vi "MSTSoftwareBin_Final.vi"() -> ()   [LabVIEW 2012]
uses:
  <vilib>/addons/database/Auxilliary.llb/DB Tools Cursor Type.ctl
  <vilib>/Utility/NIReport.llb/NI_report.lvclass
  <vilib>/addons/database/Connection.llb/DB Tools Open Connec (Path).vi
  <vilib>/addons/database/Connection.llb/Conn Execute.vi
  <vilib>/addons/database/Recordset.llb/Rec Fetch Recordset Data (R).vi
  <vilib>/addons/database/Recordset.llb/Rec Destroy - Connection.vi
  <vilib>/Utility/NIReport.llb/Append Text Table to Report (wrap).vi
  <vilib>/addons/database/_DB Variant To Data/Database Variant To Data.xnode
  <vilib>/addons/database/NI_Database_API.lvlib
  <vilib>/Utility/NIReport.llb/Excel/NI_Excel.lvclass
panel:
  out "error out":errorcluster
  out "recordset data":variant[][](array[variant])
  out "data":string
  out "appended array":string[](array[string])
  in  "Report Template":path=path "O:/Monitor/Report/MSTsoftBin.xls"
  out "Row Headers":string[](array[string])
  out "error out 2":errorcluster
  out "concatenated string":string
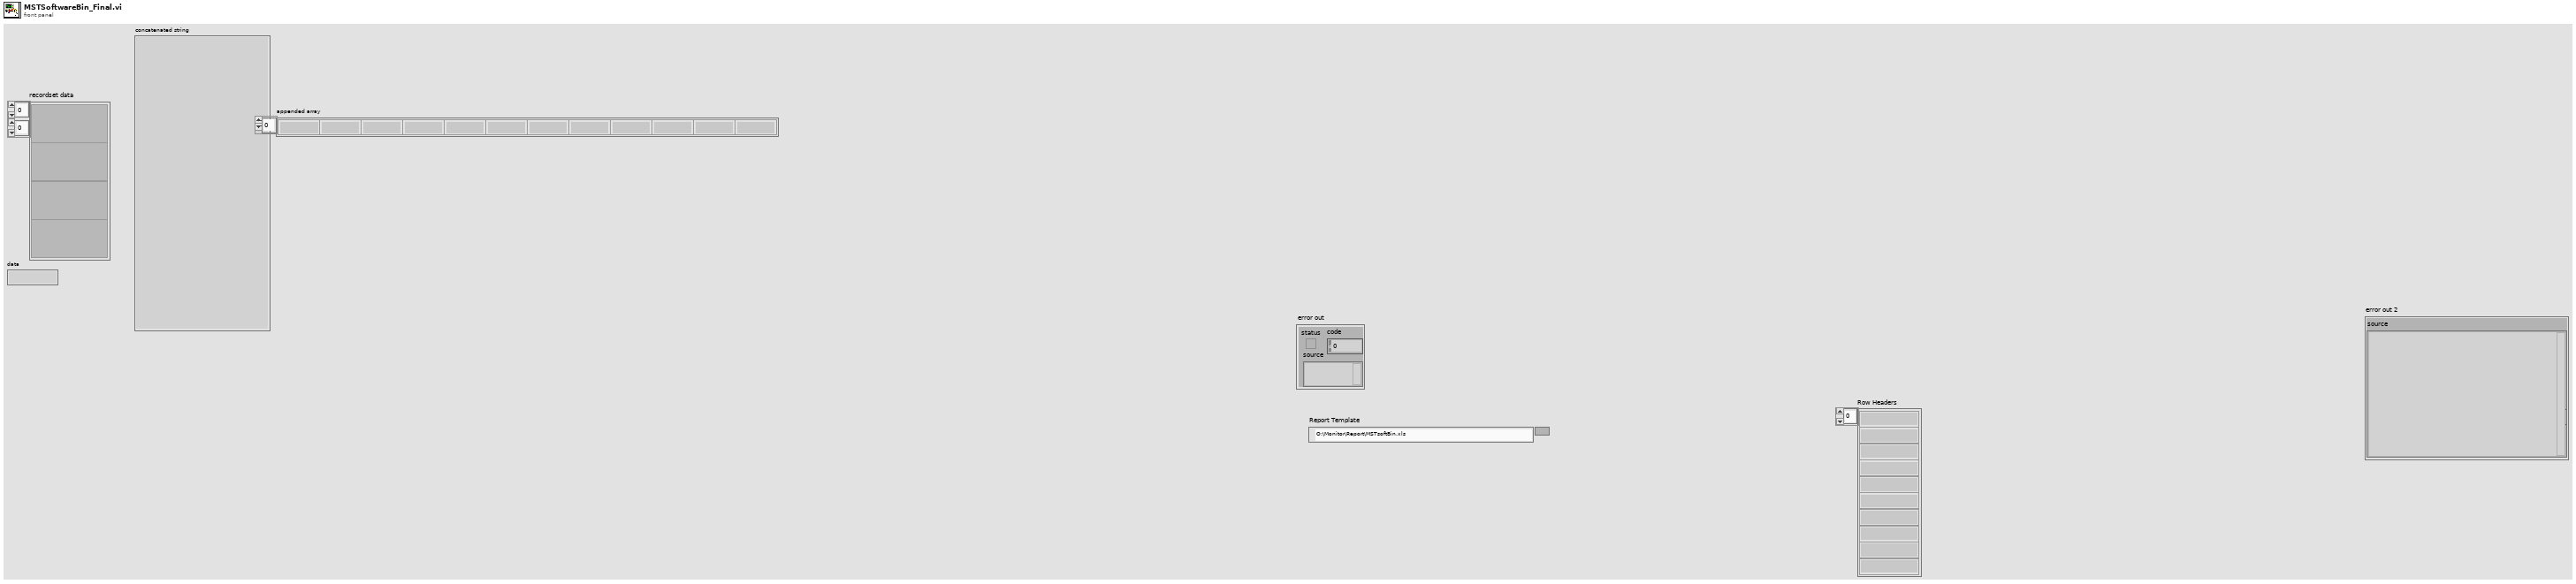
[diagram p1: front panel]
types:
  T1 = typedef "NI_Database_API.lvlib/DB Tools Cursor Type.ctl" = enum16{"forward-only", "keyset", "dynamic", "static"}
  T2 = enum16{"Standard Report", "HTML", "Word", "Excel"}
  T3 = typedef "NI_Database_API.lvlib/Conn ObjectReference.ctl" = refnum<k1>
  T4 = typedef "NI_Database_API.lvlib/Rec ObjectReference.ctl" = refnum<k1>
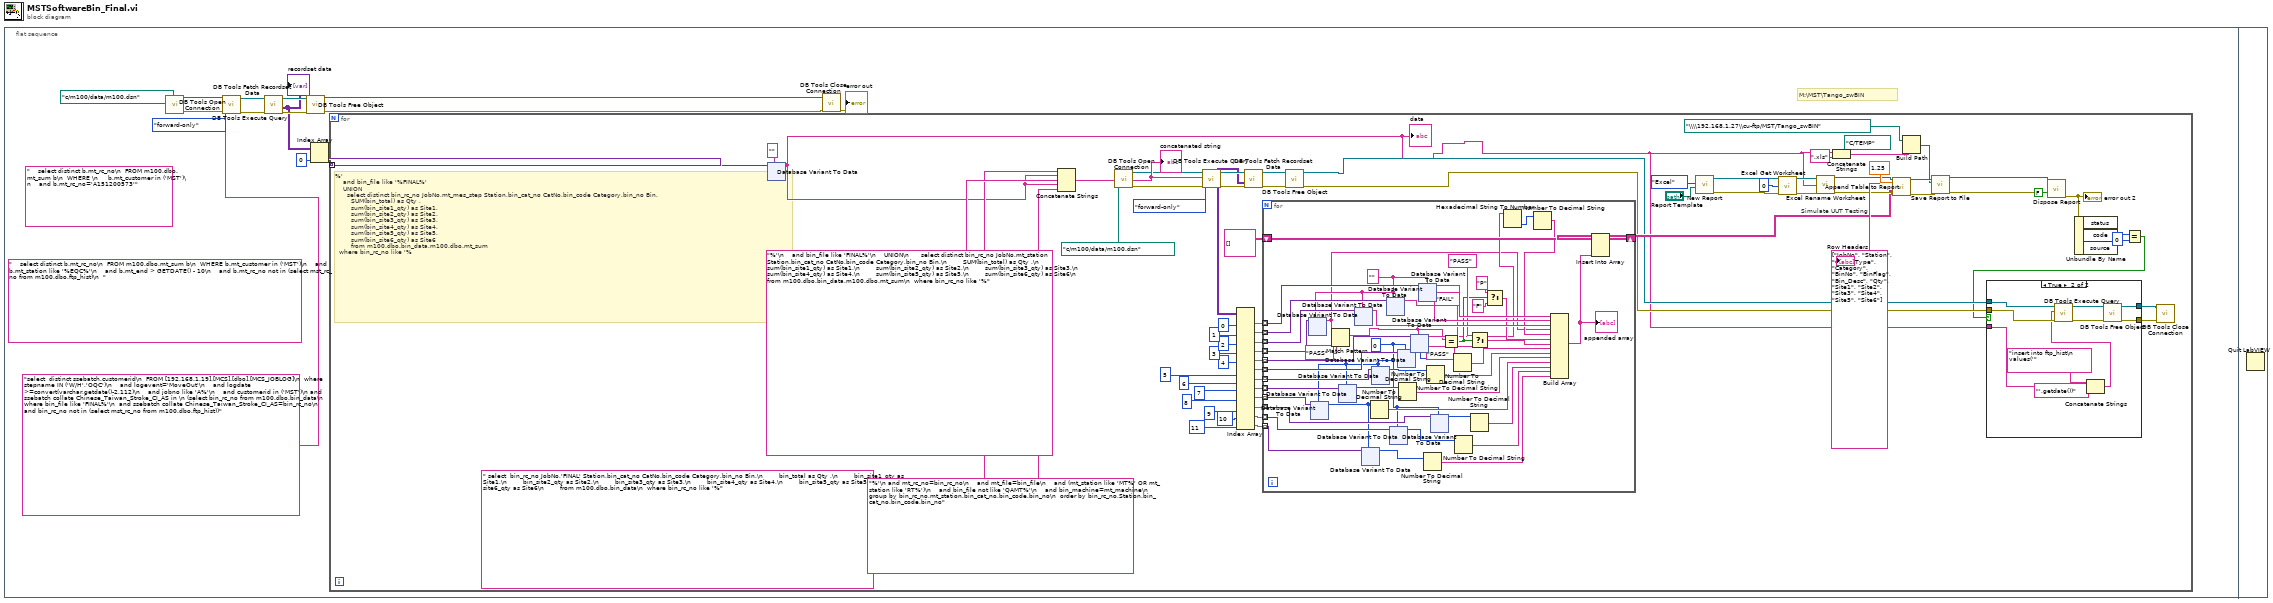
[diagram p0: block diagram]
diagram:
  n1 = flat-sequence {
    frame #0 {
      (unwired) "    select distinct b.mt_rc_no\n  FROM m100.dbo.mt_sum b\n  WHERE b.mt_customer in ('MST')\n    and b.mt_station like '%EQC%'\n    and b.mt_end > GETDATE() - 10\n    and b.mt_rc_no not in (select mst_rc_no from m100.dbo.ftp_hist)\n  " ("SQL query")
      (unwired) "    select distinct b.mt_rc_no\n  FROM m100.dbo.mt_sum b\n  WHERE \n     b.mt_customer in ('MST')\n    and b.mt_rc_no='A151200573'" ("SQL query")
      # "M:\\MST\\Tango_swBIN"
      n2 = call-poly <vilib>:"DB Tools Open Connection.vi"("connection information"=path "c:/m100/data/m100.dsn") -> ("error out"=w12:errorcluster, "connection reference"=w15:T3)  [unwired: 7 in]
      n3 = call-poly <vilib>:"DB Tools Execute Query.vi"("error in (no error)"=w12, "cursor type"=DB_Tools_Cursor_Type."forward-only", "SQL query"="select  distinct ssebatch,customerid\n  FROM [192.168.1.19].[MCS].[dbo].[MCS_JOBLOG]\n  where  stepname IN ('W/H','OQC')\n    and logevent='MoveOut'\n    and logdate >=convert(varchar,getdate()-2,112)\n    and jobno like 'A%'\n    and customerid in ('MST')\n and ssebatch collate Chinese_Taiwan_Stroke_CI_AS in \n (select bin_rc_no from m100.dbo.bin_data\n  where bin_file like 'FINAL%'\n  and ssebatch collate Chinese_Taiwan_Stroke_CI_AS=bin_rc_no\n  and bin_rc_no not in (select mst_rc_no from m100.dbo.ftp_hist))", "connection reference"=w15) -> ("error out"=w11:errorcluster, "recordset reference"=w14:T4)  [unwired: 4 in]
      n4 = call-poly <vilib>:"DB Tools Fetch Recordset Data.vi"("error in (no error)"=w11, "recordset reference"=w14) -> ("error out"=w10:errorcluster, "recordset data"=w7:variant[][], "recordset reference out"=w13:T4)  [unwired: 3 in]
      "recordset data" <- w7
      n5 = call-poly <vilib>:"DB Tools Free Object.vi"("error in (no error)"=w10, "recordset reference"=w13) -> ("error out"=w3:errorcluster, "connection reference"=w4:T3)  [unwired: 8 in]
      n6 = Index Array(array=w7, index (col)=0 ("disabled index (col)")) -> (element=w5:variant[])  [unwired: 1 in]
      n7 = for {
        tunnel: w5 -> [w85] mode=indexing
        (unwired) path "C:/TEMP" ("base path")
        # "%'\n    and bin_file like '%FINAL%'\n    UNION\n      select distinct bin_rc_no JobNo,mt_mes_step Station,bin_cat_no CatNo,bin_code Category,bin_no Bin,\n        SUM(bin_total) as Qty ,\n        sum(bin_site1_qty) as Site1,\n        sum(bin_site2_qty) as Site2,\n        sum(bin_site3_qty) as Site3,\n        sum(bin_site4_qty) as Site4,\n        sum(bin_site5_qty) as Site5,\n        sum(bin_site6_qty) as Site6\n        from m100.dbo.bin_data,m100.dbo.mt_sum\n  where bin_rc_no like '%"
        # "Simulate UUT Testing"
        n8 = xnode "Database Variant To Data"("database variant"=w85, "type"="") -> ("data"=w17:string)  [unwired: 1 in, 1 out]
        "data" <- w17
        n9 = Concatenate Strings(" select  bin_rc_no JobNo,'FINAL' Station,bin_cat_no CatNo,bin_code Category,bin_no Bin,\n        bin_total as Qty ,\n        bin_site1_qty as Site1,\n        bin_site2_qty as Site2,\n        bin_site3_qty as Site3,\n        bin_site4_qty as Site4,\n        bin_site5_qty as Site5,\n        bin_site6_qty as Site6\n        from m100.dbo.bin_data\n  where bin_rc_no like '%" ("string"), w17, "%'\n    and bin_file like 'FINAL%'\n    UNION\n      select distinct bin_rc_no JobNo,mt_station Station,bin_cat_no CatNo,bin_code Category,bin_no Bin,\n        SUM(bin_total) as Qty ,\n        sum(bin_site1_qty) as Site1,\n        sum(bin_site2_qty) as Site2,\n        sum(bin_site3_qty) as Site3,\n        sum(bin_site4_qty) as Site4,\n        sum(bin_site5_qty) as Site5,\n        sum(bin_site6_qty) as Site6\n        from m100.dbo.bin_data,m100.dbo.mt_sum\n  where bin_rc_no like '%" ("string"), w17, "%'\n and mt_rc_no=bin_rc_no\n    and mt_file=bin_file\n    and (mt_station like 'MT%' OR mt_station like 'RT%')\n    and bin_file not like 'QAMT%'\n    and bin_machine=mt_machine\n  group by bin_rc_no,mt_station,bin_cat_no,bin_code,bin_no\n  order by bin_rc_no,Station,bin_cat_no,bin_code,bin_no" ("string")) -> (w76:string)
        "concatenated string" <- w76
        n10 = call-poly <vilib>:"DB Tools Open Connection.vi"("connection information"=path "c:/m100/data/m100.dsn") -> ("error out"=w22:errorcluster, "connection reference"=w23:T3)  [unwired: 7 in]
        n11 = call-poly <vilib>:"DB Tools Execute Query.vi"("error in (no error)"=w22, "cursor type"=DB_Tools_Cursor_Type."forward-only", "SQL query"=w76, "connection reference"=w23) -> ("error out"=w81:errorcluster, "recordset reference"=w83:T4)  [unwired: 4 in]
        n12 = call-poly <vilib>:"DB Tools Fetch Recordset Data.vi"("error in (no error)"=w81, "recordset reference"=w83) -> ("error out"=w80:errorcluster, "recordset data"=w75:variant[][], "recordset reference out"=w82:T4)  [unwired: 3 in]
        n13 = Index Array(array=w75, index (col) #1=0 ("disabled index (col)"), index (col) #2=1 ("index (col)"), index (col) #3=2 ("index (col)"), index (col) #4=3 ("index (col)"), index (col) #5=4 ("index (col)"), index (col) #6=5 ("index (col)"), index (col) #7=6 ("index (col)"), index (col) #8=7 ("index (col)"), index (col) #9=8 ("index (col)"), index (col) #10=9 ("index (col)"), index (col) #11=10 ("index (col)"), index (col) #12=11 ("index (col)")) -> (element #1=w64:variant[], element #2=w63:variant[], element #3=w62:variant[], element #4=w61:variant[], element #5=w60:variant[], element #6=w59:variant[], element #7=w58:variant[], element #8=w57:variant[], element #9=w56:variant[], element #10=w55:variant[], element #11=w52:variant[], element #12=w51:variant[])  [unwired: 12 in]
        n14 = for {
          tunnel: w64 -> [w145] mode=indexing
          tunnel: w63 -> [w144] mode=indexing
          tunnel: w62 -> [w143] mode=indexing
          tunnel: w61 -> [w142] mode=indexing
          tunnel: w60 -> [w141] mode=indexing
          tunnel: w59 -> [w140] mode=indexing
          tunnel: w58 -> [w139] mode=indexing
          tunnel: w57 -> [w138] mode=indexing
          tunnel: w56 -> [w137] mode=indexing
          tunnel: w55 -> [w136] mode=indexing
          tunnel: w52 -> [w127] mode=indexing
          tunnel: w51 -> [w126] mode=indexing
          shift-right: [w121] -> w38
          shift-left: string[][] [] ("array") -> [w120]
          w112 = 0
          w135 = ""
          n15 = xnode "Database Variant To Data"("database variant"=w142, "type"=w135) -> ("data"=w100:string)  [unwired: 1 in, 1 out]
          n16 = xnode "Database Variant To Data"("database variant"=w137, "type"=w112) -> ("data"=w124:i32)  [unwired: 1 in, 1 out]
          n17 = Match Pattern(string=w100, regular expression="PASS") -> (match substring=w98:string)  [unwired: 1 in, 3 out]
          n18 = xnode "Database Variant To Data"("database variant"=w138, "type"=w112) -> ("data"=w129:i32)  [unwired: 1 in, 1 out]
          n19 = xnode "Database Variant To Data"("database variant"=w143, "type"=w135) -> ("data"=w132:string)  [unwired: 1 in, 1 out]
          n20 = xnode "Database Variant To Data"("database variant"=w126, "type"=w124) -> ("data"=w125:i32)  [unwired: 1 in, 1 out]
          n21 = Number To Decimal String(number=w124) -> (decimal integer string=w116:string)  [unwired: 1 in]
          n22 = xnode "Database Variant To Data"("database variant"=w139, "type"=w112) -> ("data"=w130:i32)  [unwired: 1 in, 1 out]
          n23 = xnode "Database Variant To Data"("database variant"=w144, "type"=w135) -> ("data"=w133:string)  [unwired: 1 in, 1 out]
          n24 = xnode "Database Variant To Data"("database variant"=w127, "type"=w112) -> ("data"=w123:i32)  [unwired: 1 in, 1 out]
          n25 = xnode "Database Variant To Data"("database variant"=w140, "type"=w112) -> ("data"=w131:i32)  [unwired: 1 in, 1 out]
          n26 = Number To Decimal String(number=w129) -> (decimal integer string=w115:string)  [unwired: 1 in]
          n27 = xnode "Database Variant To Data"("database variant"=w141, "type"=w98) -> ("data"=w102:string)  [unwired: 1 in, 1 out]
          n28 = xnode "Database Variant To Data"("database variant"=w145, "type"=w135) -> ("data"=w134:string)  [unwired: 1 in, 1 out]
          n29 = Number To Decimal String(number=w125) -> (decimal integer string=w119:string)  [unwired: 1 in]
          n30 = Number To Decimal String(number=w130) -> (decimal integer string=w114:string)  [unwired: 1 in]
          n31 = xnode "Database Variant To Data"("database variant"=w136, "type"=w112) -> ("data"=w128:i32)  [unwired: 1 in, 1 out]
          n32 = Equal?(x=w98, y="PASS") -> (x = y?=w108:bool)
          n33 = Number To Decimal String(number=w131) -> (decimal integer string=w113:string)  [unwired: 1 in]
          n34 = Number To Decimal String(number=w123) -> (decimal integer string=w118:string)  [unwired: 1 in]
          n35 = Number To Decimal String(number=w128) -> (decimal integer string=w117:string)  [unwired: 1 in]
          n36 = Select(t="PASS", s=w108, f="FAIL") -> (s? t:f=w109:string)
          n37 = Select(t="P", s=w108, f="F") -> (s? t:f=w105:string)
          n38 = Hexadecimal String To Number(string=w102) -> (number=w103:u32)  [unwired: 2 in, 1 out]
          n39 = Number To Decimal String(number=w103) -> (decimal integer string=w101:string)  [unwired: 1 in]
          n40 = Build Array(w134, w133, w132, w100, w101, w105, w109, w113, w114, w115, w116, w117, w118, w119) -> (w122:string[])
          "appended array" <- w122
          n41 = Insert Into Array(array=w120, new element=w122) -> (w121:string[][])  [unwired: 2 in]
        }
        n42 = call-poly <vilib>:"DB Tools Free Object.vi"("error in (no error)"=w80, "recordset reference"=w82) -> ("error out"=w27:errorcluster, "connection reference"=w28:T3)  [unwired: 8 in]
        n43 = call <vilib>:"New Report.vi"("report type"=T2."Excel" ("Report Type"), "template (empty)"="Report Template") -> ("report out"=w45:refnum<class "NI_report.lvclass">, "error out"=w44:errorcluster)  [unwired: 12 in]
        n44 = call <vilib>:"Excel Get Worksheet.vi"("report in"=w45, "worksheet index (0)"=0, "error in (no error)"=w44) -> ("report out"=w42:refnum<class "NI_report.lvclass">, "error out"=w40:errorcluster)  [unwired: 11 in]
        n45 = call <vilib>:"Excel Rename Worksheet.vi"("report in"=w42, "worksheet name (\"\")"=w17, "error in (no error)"=w40) -> ("report out"=w41:refnum<class "NI_report.lvclass">, "error out"=w39:errorcluster)  [unwired: 11 in]
        n46 = Concatenate Strings(w17, ".xls" ("string")) -> (w31:string)
        n47 = call-poly <vilib>:"Append Table to Report.vi"("report in"=w41, "column width (1)"=1.25, "column headers"=string[] ["JobNo", "Station", "CatNo Type", "Category", "BinNo", "BinFlag", "Bin_Desc", "Qty", "Site1", "Site2", "Site3", "Site4", "Site5", "Site6"] ("row headers"), "text data"=w38, "error in (no error)"=w39) -> ("report out"=w34:refnum<class "NI_report.lvclass">, "error out"=w33:errorcluster)  [unwired: 7 in, 2 out]
        n48 = Build Path(base path=path "\\\\192.168.1.27\\cu-ftp/MST/Tango_swBIN", name or relative path=w31) -> (appended path=w30:path)
        n49 = call-dynamic "Save Report to File.vi"("report in"=w34, "report file path"=w30, "error in (no error)"=w33) -> ("report out"=w36:refnum<class "NI_report.lvclass">, "error out"=w35:errorcluster)  [unwired: 11 in]
        n50 = call-dynamic "Dispose Report.vi"("report in"=w36, "save changes? (F)"=FALSE, "error in (no error)"=w35) -> ("error out"=w29:errorcluster)  [unwired: 12 in]
        "error out 2" <- w29
        n51 = Unbundle By Name(w29) -> ("code"=w26:i32)  [unwired: 2 out]
        n52 = Equal?(x=w26, y=0) -> (x = y?=w24:bool)
        n53 = case shown="True" w24 {
          tunnel: w28 -> [w87 w97]
          tunnel: w27 -> [w86 w96]
          tunnel: w17 -> [_ w94]
          tunnel: [w87 w89] -> w20
          tunnel: [w86 w88] -> w19
          frame False {
          }
          frame True {
            n54 = Concatenate Strings("insert into ftp_hist\n values('" ("string"), w94, "',getdate())" ("string")) -> (w92:string)
            n55 = call-poly <vilib>:"DB Tools Execute Query.vi"("error in (no error)"=w96, "SQL query"=w92, "connection reference"=w97) -> ("error out"=w90:errorcluster, "recordset reference"=w91:T4)  [unwired: 5 in]
            n56 = call-poly <vilib>:"DB Tools Free Object.vi"("error in (no error)"=w90, "recordset reference"=w91) -> ("error out"=w88:errorcluster, "connection reference"=w89:T3)  [unwired: 8 in]
          }
        }
        n57 = call <vilib>:"DB Tools Close Connection.vi"("error in (no error)"=w19, "connection reference"=w20) -> ()  [unwired: 5 in, 1 out]
      }
      n58 = call <vilib>:"DB Tools Close Connection.vi"("error in (no error)"=w3, "connection reference"=w4) -> ("error out"=→"error out":errorcluster)  [unwired: 5 in]
    }
    frame #1 {
      n59 = Quit LabVIEW() -> ()  [unwired: 1 in]
    }
  }
